vi "Shell f.vi"(11 "Reynolds Number":dbl) -> (3 "Numeric":dbl)   [LabVIEW 2019]
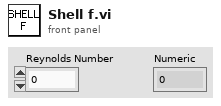
[diagram p1: front panel]
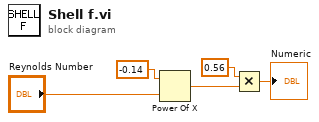
[diagram p0: block diagram]
diagram:
  n1 = Power Of X(1:"Reynolds Number", 2:-0.14 ("y")) -> (0:w3:dbl)
  n2 = Multiply(x=0.56, y=w3) -> (x*y=→"Numeric":dbl)
